vi "createSerialProtocol.vi"(8 "error in (no error)":errorcluster, 9 "simulateSerialData":refnum<class "SimulateSerialData.lvclass">, 10 "Serial Protocol":T1, 11 "SerialCommFactory in":refnum<class "SerialProtocolFactory.lvclass">) -> (0 "error out":errorcluster, 2 "serialProtocol":refnum<class "SerialProtocol.lvclass">, 3 "SerialCommFactory out":refnum<class "SerialProtocolFactory.lvclass">)   [LabVIEW 2013, in "SerialProtocols.lvlib" / "SerialProtocolFactory.lvclass"]
uses:
  <userlib>/Common/SerialProtocols/SerialProtocolFactory/SerialProtocolFactory/SerialProtocolFactory.lvclass
  <userlib>/Common/SerialProtocols/SerialProtocol/RS485/RS485.lvclass
  <userlib>/Common/SerialProtocols/SerialProtocol/RS232/RS232.lvclass
  <userlib>/Common/SerialProtocols/SerialProtocol/SerialSimulator/SerialSimulator.lvclass
  <userlib>/Common/SerialProtocols/Configuration/SerialProtocol.ctl
  <userlib>/Common/SerialProtocols/SerialProtocols.lvlib
  <userlib>/Common/SerialProtocols/SerialProtocol/SerialProtocol/SerialProtocol.lvclass
  LSST_TS/SystemSW/M2AADT/SimulateSerialData/SimulateSerialData/SimulateSerialData.lvclass
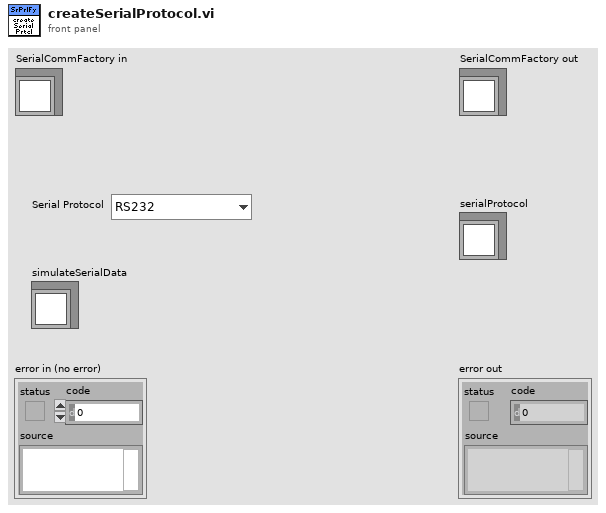
[diagram p1: front panel]
types:
  T1 = typedef "SerialProtocols.lvlib/SerialProtocol.ctl" = enum16{"RS232", "RS485", "SerialSimulator"}
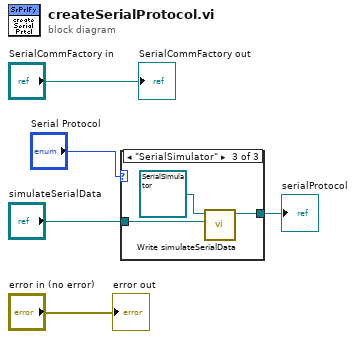
[diagram p0: block diagram]
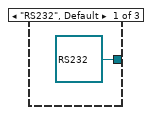
[diagram p2: hidden frame]
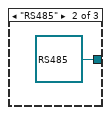
[diagram p3: hidden frame]
diagram:
  n1 = case shown="\"SerialSimulator\"" "Serial Protocol" {
    tunnel: [refnum<class "RS232.lvclass"> refnum ("RS232.lvclass") refnum<class "RS485.lvclass"> refnum ("RS485.lvclass") w8] -> w4
    tunnel: "simulateSerialData" -> [_ _ w10]
    frame "RS232", Default {
    }
    frame "RS485" {
    }
    frame "SerialSimulator" {
      n2 = call <userlib>:"Write simulateSerialData.vi"("simulateSerialData"=w10, "SerialSimulator in"=refnum<class "SerialSimulator.lvclass"> refnum ("SerialSimulator.lvclass")) -> ("SerialSimulator out"=w8:refnum<class "SerialSimulator.lvclass">)  [unwired: 9 in]
    }
  }
  "serialProtocol" <- w4
  "error out" <- "error in (no error)"
  "SerialCommFactory out" <- "SerialCommFactory in"
